vi "WriteRead.vi"(8 "error in (no error)":errorcluster, 9 "write buffer":string, 10 "Data in":string[](array[string]), 11 "VISA Refnum in":refnum<visa-resource-name>) -> (0 "error out":errorcluster, 2 "Data out":string[](array[string]), 3 "VISA resource name out":refnum<visa-resource-name>)   [LabVIEW 2020]
panel:
  in  "stop":bool
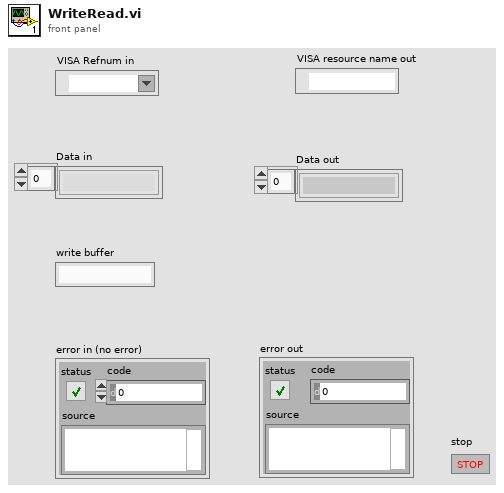
[diagram p1: front panel]
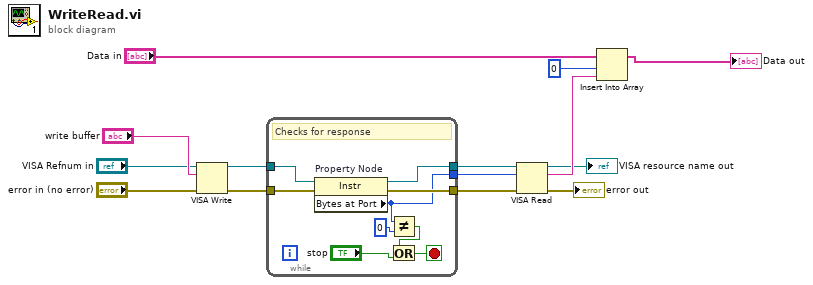
[diagram p0: block diagram]
diagram:
  n1 = VISA Write(VISA resource name="VISA Refnum in", write buffer="write buffer", error in (no error)="error in (no error)") -> (VISA resource name out=w5:refnum<visa-resource-name>, error out=w4:errorcluster)  [unwired: 1 out]
  n2 = while {
    tunnel: w5 -> [w22]
    tunnel: w4 -> [w21]
    tunnel: [w20] -> w3
    tunnel: [w19] -> w2
    tunnel: [w18] -> w1
    stop <- w17 stop-if-true
    # "Checks for response"
    n3 = property on="Property Node" class="Instr"(reference=w22, error in=w21) -> (reference out=w19:refnum<visa-resource-name>, error out=w20:errorcluster, "Bytes at Port"=w18:u32)
    n4 = Not Equal?(x=w18, y=u32 0) -> (x != y?=w15:bool)
    n5 = Or(x=w15, y="stop") -> (x .or. y?=w17:bool)
  }
  n6 = VISA Read(VISA resource name=w2, byte count=w1, error in (no error)=w3) -> (VISA resource name out=→"VISA resource name out":refnum<visa-resource-name>, read buffer=w12:string, error out=→"error out":errorcluster)  [unwired: 1 out]
  n7 = Insert Into Array "Insert Into Array"(array="Data in", index=0, new element=w12) -> (→"Data out":string[])
